vi "Write.vi"(8 "error in (no error)":errorcluster, 9 "write enable":bool=TRUE, 11 "ICPCON ET7024 in":refnum<class "SHINI SHD.lvclass">) -> (0 "error out":errorcluster, 3 "ICPCON ET7024 out":refnum<class "SHINI SHD.lvclass">)   [LabVIEW 2021]
uses:
  Master CR.lvclass
  SHINI SHD.lvclass
  D:/my_projects/projects/21/Master CR/Master CR.lvclass
  D:/my_projects/projects/21/Master CR/Devices/ET7000/TCP/TCP.lvclass
  Modbus_v121c/Network Protocol/Network Master/Network Master.lvclass
  ET7000/TCP/TCP.lvclass
  Modbus_v121c/Data Model/Device Data Model.lvclass
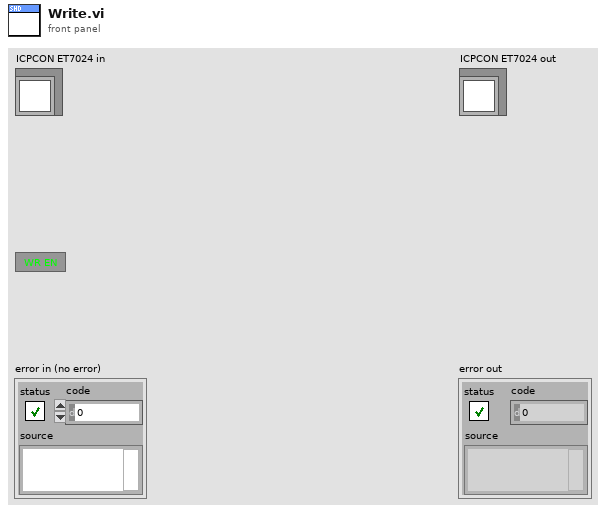
[diagram p1: front panel]
types:
  T1 = typedef "Device Data Model.lvclass/N channel.ctl" = cluster{"N DI channel":i32, "N DO channel":i32, "N AI channel":i32, "N AO channel":i32}
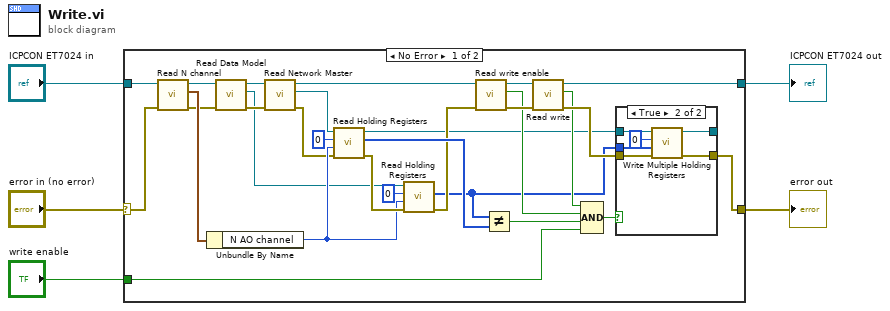
[diagram p0: block diagram]
diagram:
  n1 = case shown="No Error" "error in (no error)" {
    selector: "error in (no error)" -> [w30 w44]
    tunnel: [w6 w44] -> w3
    tunnel: [w14 w43] -> w4
    tunnel: "ICPCON ET7024 in" -> [w32 w43]
    tunnel: "write enable" -> [w16 _]
    frame No Error {
      n2 = call "Read N channel.vi"("error in (no error)"=w30, "Master CR in"=w32) -> ("error out"=w29:errorcluster, "N channel"=w33:T1, "Master CR out"=w31:refnum<class "SHINI SHD.lvclass">)  [unwired: 7 in]
      n3 = Unbundle By Name(w33) -> ("N AO channel"=w19:i32)
      n4 = call "Read Data Model.vi"("error in (no error)"=w29, "Master CR in"=w31) -> ("error out"=w12:errorcluster, "Data Model"=w8:refnum<class "Device Data Model.lvclass">, "Master CR out"=w13:refnum<class "SHINI SHD.lvclass">)  [unwired: 7 in]
      n5 = call "Read Network Master.vi"("error in (no error)"=w12, "TCP in"=w13) -> ("error out"=w7:errorcluster, "Network Master"=w9:refnum<class "Network Master.lvclass">, "TCP out"=w10:refnum<class "SHINI SHD.lvclass">)  [unwired: 7 in]
      n6 = call "Read Holding Registers.vi"("error in (no error)"=w7, "number of holding registers"=w19, "starting address"=u16 0, "Modbus master in"=w9) -> ("error out"=w20:errorcluster, "register values"=w22:u16[], "Modbus master out"=w11:refnum<class "Network Master.lvclass">)  [unwired: 5 in]
      n7 = call-dynamic "Read Holding Registers.vi"("error in"=w20, "number of registers"=w19, "starting address"=u16 0, "device data model in"=w8) -> ("error out"=w21:errorcluster, "data"=w15:u16[])  [unwired: 5 in, 1 out]
      n8 = call "Read write enable.vi"("error in (no error)"=w21, "Master CR in"=w10) -> ("error out"=w26:errorcluster, "write enable"=w17:bool, "Master CR out"=w27:refnum<class "SHINI SHD.lvclass">)  [unwired: 7 in]
      n9 = Not Equal?(x=w15, y=w22) -> (x != y?=w28:bool)
      n10 = call "Read write.vi"("error in (no error)"=w26, "Master CR in"=w27) -> ("error out"=w25:errorcluster, "Write"=w18:bool, "Master CR out"=w14:refnum<class "SHINI SHD.lvclass">)  [unwired: 7 in]
      n11 = Compound Arithmetic op=AND(w18, w17, w28, w16) -> (w34:bool)
      n12 = case shown="True" w34 {
        tunnel: w25 -> [w36 w41]
        tunnel: [w36 w39] -> w6
        tunnel: w15 -> [_ w40]
        tunnel: [w35 w38] -> _
        tunnel: w11 -> [w35 w37]
        frame False {
        }
        frame True {
          n13 = call "Write Multiple Holding Registers.vi"("error in (no error)"=w41, "holding register values"=w40, "starting address"=u16 0, "Modbus master in"=w37) -> ("error out"=w39:errorcluster, "Modbus master out"=w38:refnum<class "Network Master.lvclass">)  [unwired: 6 in]
        }
      }
    }
    frame Error {
    }
  }
  "error out" <- w3
  "ICPCON ET7024 out" <- w4
